vi "2023 Gripper Control.vi"(1 "Button 6":bool, 2 "Button 5":bool) -> (0 "Numeric":dbl)   [LabVIEW 2020]
uses:
  <vilib>/Rock Robotics/WPI/ThirdParty/REV Robotics/REVLib/Typedef/Spark MAX Control Type.ctl
panel:
  # "I've got the velocity for the motor set at 0.8.\nI'm hopful that I'm using the motor correctly\nsince I set the motor type to 'brushed' when\nI configured the motor controller."
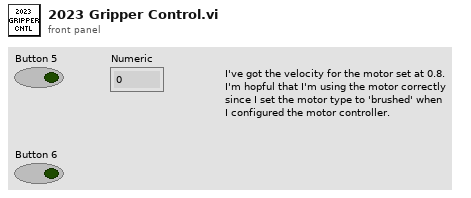
[diagram p1: front panel]
types:
  T1 = typedef "Spark MAX Control Type.ctl" = enum16{"Percent VBus", "Voltage", "Velocity", "Position", "Smart Motion", "Current", "Smart Velocity"}
  T2 = typedef "WPI_MotorControlDeviceRef.ctl" = cluster{"DeviceStatus":errorcluster, "Type":T3, "PWM":cluster{"PWM Channel":T4, "DeadBand":T5}, "CAN":cluster{"Device Number":u8, "SetOutput VI Ref":variant, "GetOutput VI Ref":variant, "Enable VI Ref":variant, "Disable VI Ref":variant, "Data":variant}, "Invert":bool, "DIO PWM":cluster{"PWM \"Enable\" Channel":T4, "DIOChannel":T6, "PWM Rate":dbl}}
  T3 = typedef "WPI_MotorControlType.ctl" = enum16{"PWM", "CAN", "DIO PWM"}
  T4 = typedef "FPGA_DIOPWMChannel.ctl" = enum8{"PWM 0", "PWM 1", "PWM 2", "PWM 3", "PWM 4", "PWM 5", "PWM 6", "PWM 7", "PWM 8", "PWM 9", "PWM MXP 0", "PWM MXP 1", "PWM MXP 2", "PWM MXP 3", "PWM MXP 4", "PWM MXP 5", "PWM MXP 6", "PWM MXP 7", "PWM MXP 8", "PWM MXP 9", "Invalid"}
  T5 = typedef "WPI_PWMDeadband.ctl" = cluster{"Name":string, "maxPositivePwm":i32, "minPositivePwm":i32, "centerPwm":i32, "maxNegativePwm":i32, "minNegativePwm":i32, "angularRange":u16}
  T6 = typedef "FPGA_DIOChannel.ctl" = enum8{"DIO 0", "DIO 1", "DIO 2", "DIO 3", "DIO 4", "DIO 5", "DIO 6", "DIO 7", "DIO 8", "DIO 9", "DIO MXP 0", "DIO MXP 1", "DIO MXP 2", "DIO MXP 3", "DIO MXP 4", "DIO MXP 5", "DIO MXP 6", "DIO MXP 7", "DIO MXP 8", "DIO MXP 9", "DIO MXP 10", "DIO MXP 11", "DIO MXP 12", "DIO MXP 13", "DIO MXP 14", "DIO MXP 15", "SPI Port CS1", "SPI Port CS2", "SPI Port CS3", "SPI Port MISO", "SPI Port MOSI", "Invalid"}
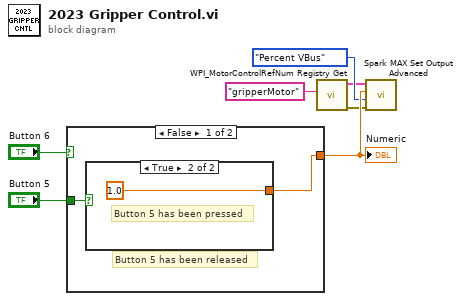
[diagram p0: block diagram]
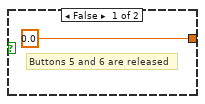
[diagram p2: hidden frame]
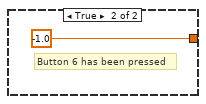
[diagram p3: hidden frame]
diagram:
  n1 = case shown="False" "Button 6" {
    tunnel: [w8 -1.0] -> w7
    tunnel: "Button 5" -> [w9 _]
    frame False {
      # "Button 5 has been released"
      n2 = case shown="True" w9 {
        tunnel: [0.0 1.0] -> w8
        frame False {
          # "Buttons 5 and 6 are released"
        }
        frame True {
          # "Button 5 has been pressed"
        }
      }
    }
    frame True {
      # "Button 6 has been pressed"
    }
  }
  "Numeric" <- w7
  n3 = call <vilib>:"WPI_MotorControlRefNum Registry Get.vi"("refnum name"="gripperMotor") -> ("error out"=w3:errorcluster, "MotorControlDevRef"=w2:T2)  [unwired: 9 in]
  n4 = call <vilib>:"Spark MAX Set Output Advanced.vi"("error in (no error)"=w3, "Control Mode"=Spark_MAX_Control_Type."Percent VBus", "Setpoint"=w7, "MotorControlDevRef"=w2) -> ()  [unwired: 6 in, 2 out]
